vi "DD Test Subject.vi"   [LabVIEW 2011]
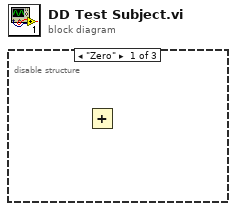
[diagram p0: block diagram]
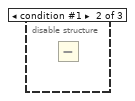
[diagram p2: hidden frame]
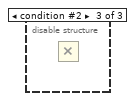
[diagram p3: hidden frame]
diagram:
  n1 = disable-structure shown="\"Zero\"" {
    frame condition #0 (active) {
      n2 = Add() -> ()  [unwired: 2 in, 1 out]
    }
    frame condition #1 {
      n3 = Subtract() -> ()  [unwired: 2 in, 1 out]
    }
    frame condition #2 {
      n4 = Multiply() -> ()  [unwired: 2 in, 1 out]
    }
  }
